vi "Construct.vi"(1 "Canvas Ref in":refnum<vi>, 2 "Background Color in":u32(colorbox)) -> (0 "Drawing System out":refnum<class "DrawingSystem.lvclass">)   [LabVIEW 2022 SP3, in "DrawingSystem.lvclass"]
uses:
  DrawingSystem.lvclass
  DrawingSystem.lvclass/DrawingSystem.ctl
  Math/Vector2/Vector2.lvclass
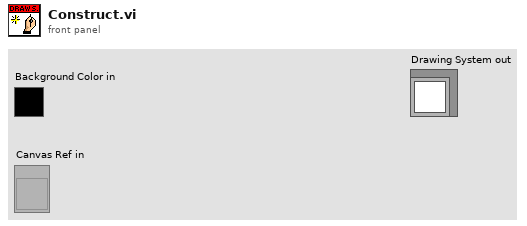
[diagram p1: front panel]
types:
  T1 = typedef "LVBoundsTypeDef.ctl" = cluster{"Width":u32, "Height":u32}
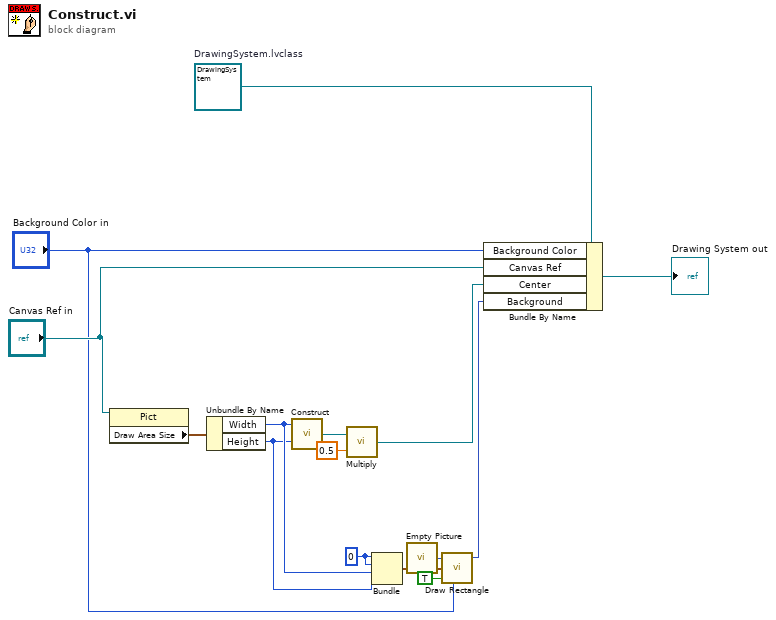
[diagram p0: block diagram]
diagram:
  w5 = 0
  w15 = refnum<class "DrawingSystem.lvclass"> refnum  # DrawingSystem.lvclass
  n1 = property class="Pict"(reference="Canvas Ref in") -> ("Draw Area Size"=w12:T1)  [unwired: 1 in, 2 out]
  n2 = Unbundle By Name(w12) -> ("Width"=w3:u32, "Height"=w2:u32)
  n3 = call "Construct.vi"("y"=w2, "x"=w3) -> ("Vec2 out"=w11:refnum<class "Vector2.lvclass">)
  n4 = call "Multiply.vi"("Scalar"=0.5, "Vector in"=w11) -> ("Vector out"=w9:refnum<class "Vector2.lvclass">)
  n5 = Bundle(w5, w5, "Width"=w3, "Height"=w2) -> (w6:cluster{i32, i32, "Width":u32, "Height":u32})  [unwired: 1 in]
  n6 = call "Empty Picture"() -> ("empty picture"=w8:picture)
  n7 = call <vilib>:"Draw Rectangle.vi"("picture"=w8, "rect"=w6, "fill?(F)"=TRUE, "color(black)"="Background Color in") -> ("new picture"=w1:picture)  [unwired: 5 in]
  n8 = Bundle By Name(cluster=w15, "Background Color"="Background Color in", "Canvas Ref"="Canvas Ref in", "Center"=w9, "Background"=w1) -> (→"Drawing System out":refnum<class "DrawingSystem.lvclass">)
